vi "getNext.vi"(8 "error in (no error)":errorcluster, 11 "LLNode in":refnum<class "LLNode.lvclass">) -> (0 "error out":errorcluster, 2 "next":refnum<data-value>, 3 "LLNode out":refnum<class "LLNode.lvclass">)   [LabVIEW 2010, in "LLNode.lvclass"]
doc: "Gets the node next in the list."
uses:
  LLNode.lvclass
  LLNode.lvclass/LLNode.ctl
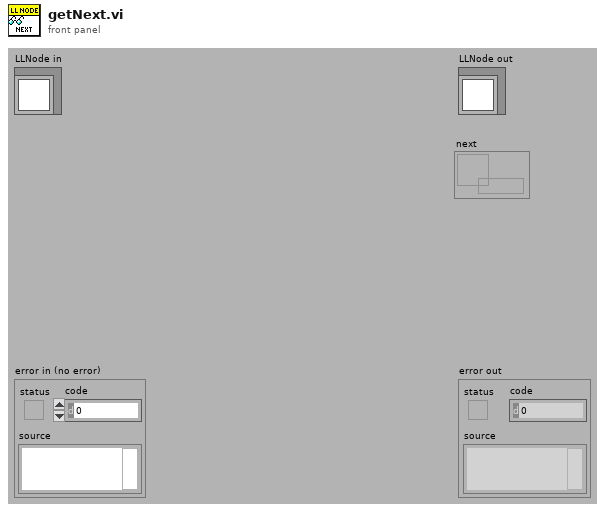
[diagram p1: front panel]
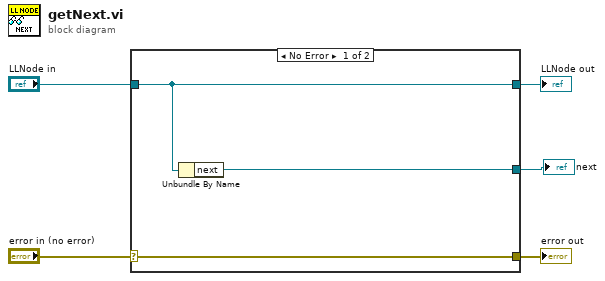
[diagram p0: block diagram]
diagram:
  n1 = case shown="No Error" "error in (no error)" {
    selector: "error in (no error)" -> [w8 w9]
    tunnel: [w8 w9] -> w4
    tunnel: [w7 w10] -> w2
    tunnel: "LLNode in" -> [w7 w10]
    tunnel: [w6 _] -> w1
    frame No Error {
      n2 = Unbundle By Name(w7) -> ("next"=w6:refnum<data-value>)
    }
    frame Error {
    }
  }
  "error out" <- w4
  "LLNode out" <- w2
  "next" <- w1
